vi "AT_Pro Main.vi"() -> ()   [LabVIEW 2018]
doc: "This template is for the Queued Message Handler design pattern.\n\nThe Event Handling Loop generates messages based on user interface actions.\n\nThe Message Handling Loop processes messages generated by the Event Handling Loop, or by other messages. The messages are string values, so new messages can be added easily to the Message Cases case structure in the Message Handling Loop. Each message cluster can also provide an optional value for Message Data, which is a variant that can be converted to whatever message-specific data is required."
uses:
  controls/AT_Pro UI Data.ctl
  <vilib>/DAQmx/read.llb/DAQmx Read (Analog 2D DBL NChan NSamp).vi
  support/Message Queue/Enqueue Message (Array).vi
  support/Message Queue/Enqueue Message (Single).vi
  <vilib>/DAQmx/miscellaneous.llb/DAQmx Fill In Error Info.vi
  <vilib>/Utility/error.llb/Error Cluster From Error Code.vi
  <vilib>/ErrorRing/Error Ring.xnode
  support/Message Queue/AT_Pro Message Queue.lvlib
  support/User Event - Stop/AT_Pro User Event - Stop.lvlib
panel:
  out "read buffer":string
  out "Waveform Graph":dbl[][](graph)
  in  "DAQmx Channel":tag="cDAQ1Mod4/ai17, cDAQ1Mod4/ai19"
  in  "COM Port":refnum<visa-resource-name>="COM8"
  in  "Stop Measure":bool
  in  "Start Measure":bool
  in  "Exit":bool
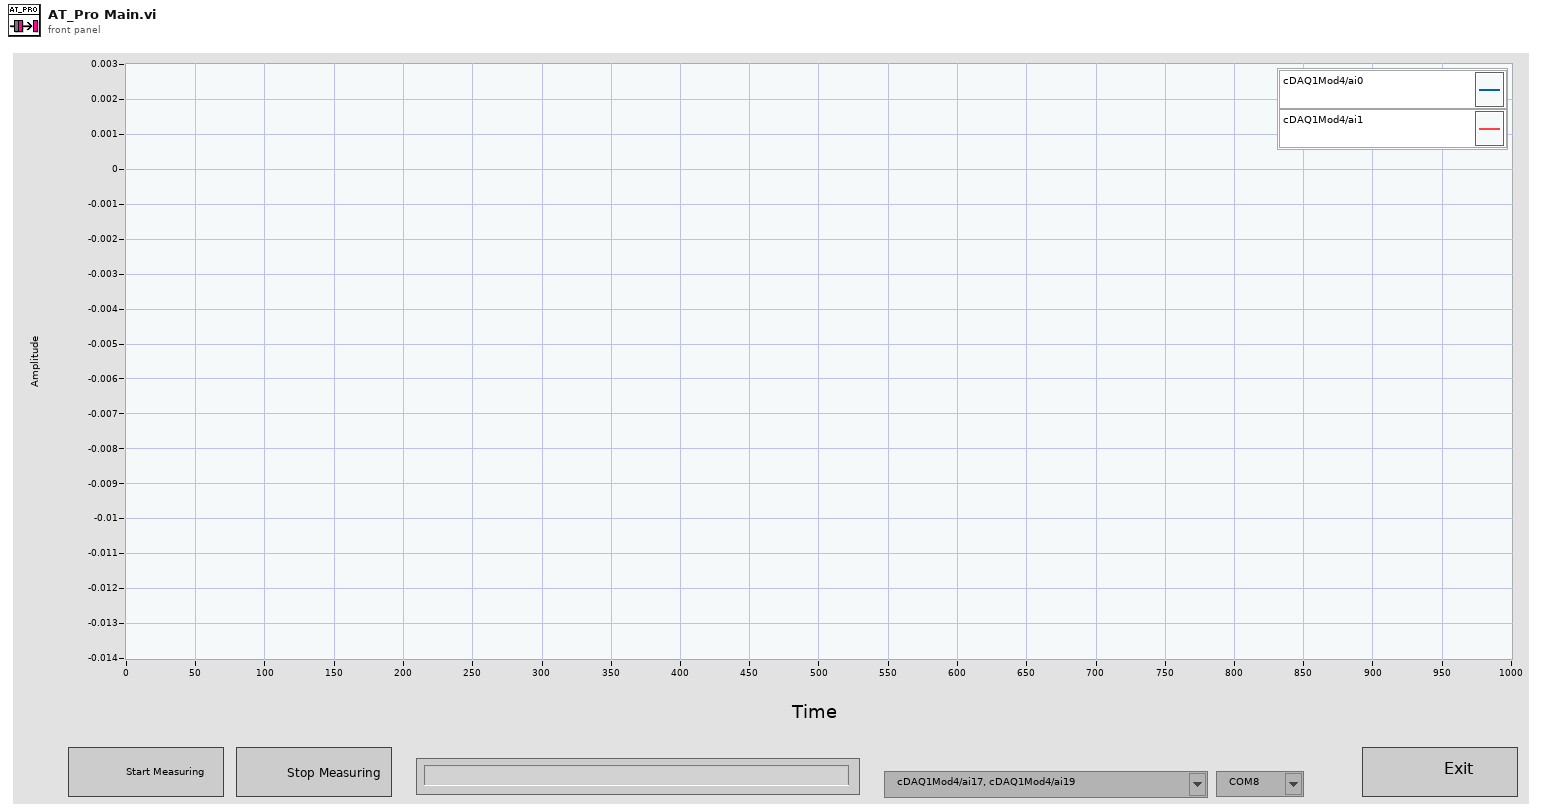
[diagram p1: front panel]
types:
  T1 = typedef "AT_Pro UI Data.ctl" = cluster{"Do Something Ref":refnum<vi>, "Do Something Else Ref":refnum<vi>, "Exit Button Ref":refnum<vi>, "Chart Refnum":refnum<vi>, "COM Port":refnum<visa-resource-name>, "DAQmx Ref":refnum<k21>}
  T2 = typedef "AT_Pro Message Queue.lvlib/All Message Queues.ctl" = cluster{"UI":refnum<queue>}
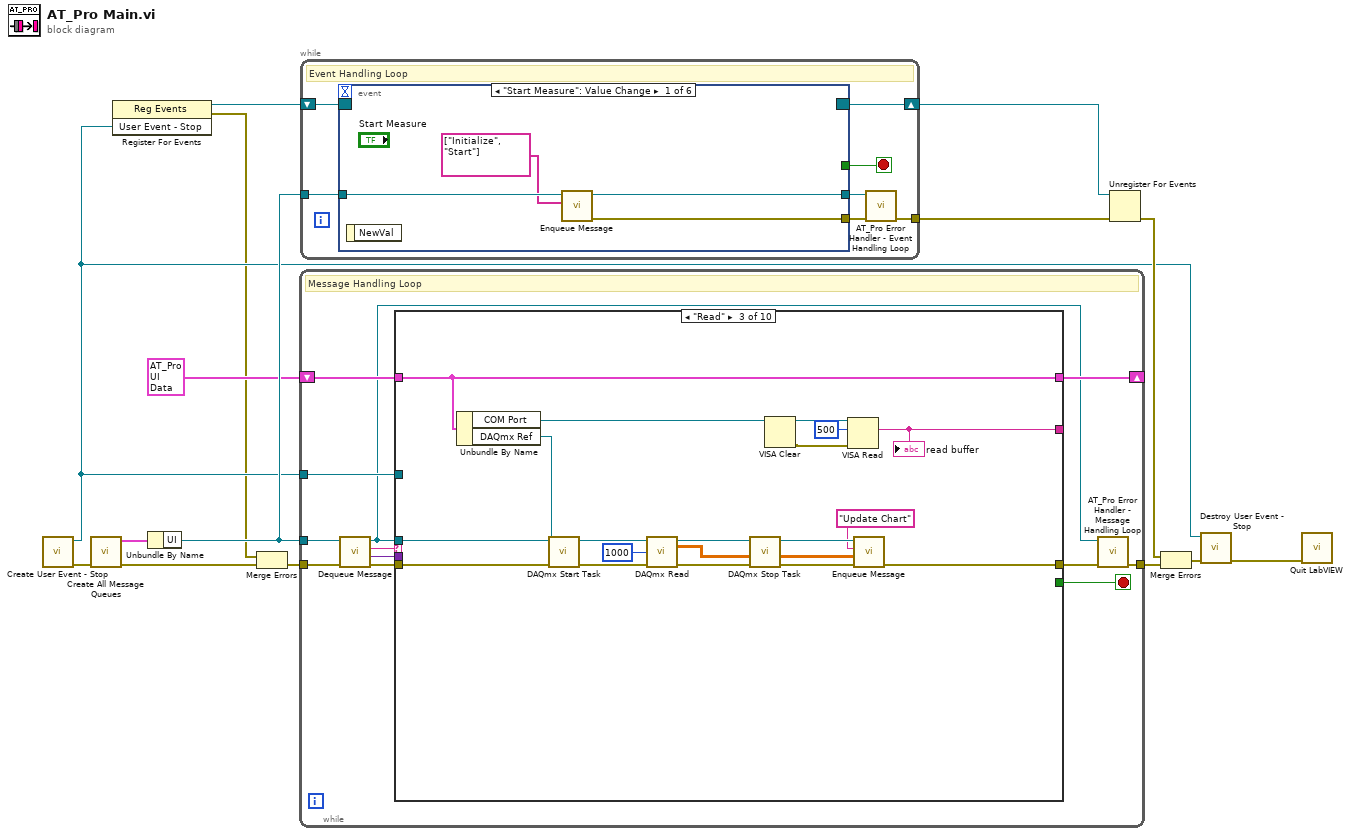
[diagram p0: block diagram]
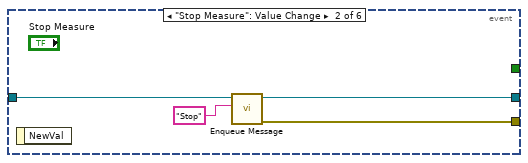
[diagram p2: hidden frame]
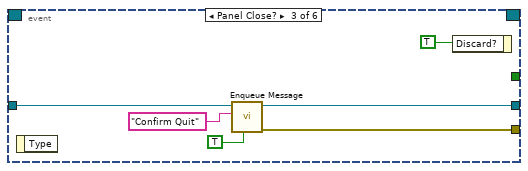
[diagram p3: hidden frame]
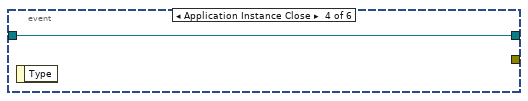
[diagram p4: hidden frame]
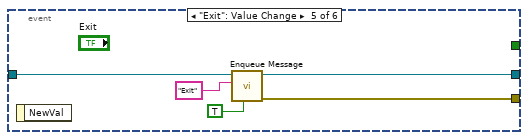
[diagram p5: hidden frame]
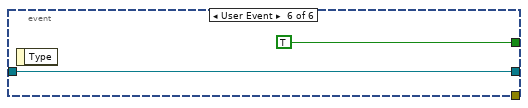
[diagram p6: hidden frame]
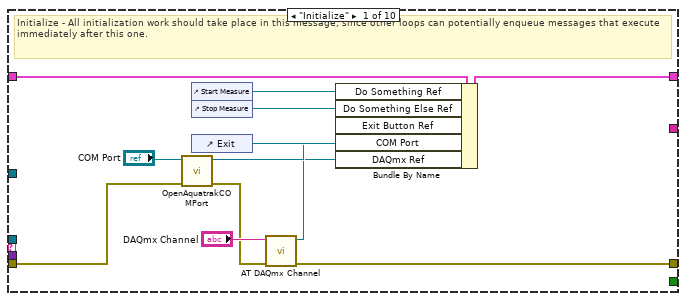
[diagram p7: hidden frame]
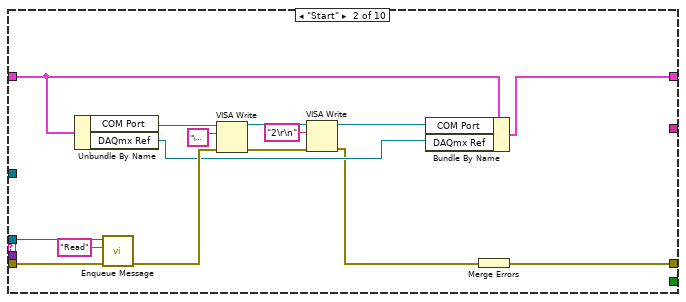
[diagram p8: hidden frame]
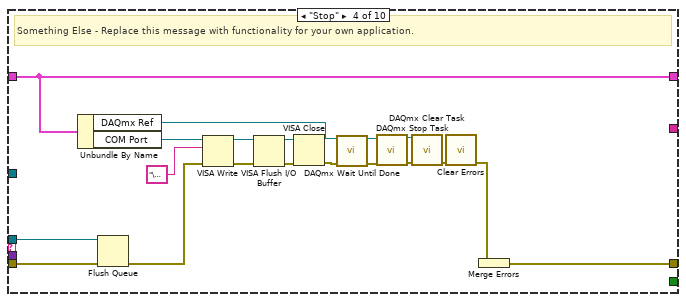
[diagram p9: hidden frame]
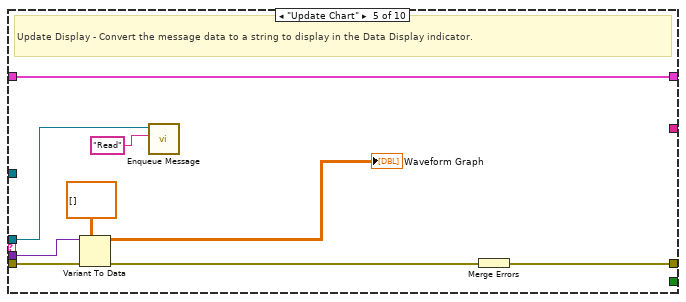
[diagram p10: hidden frame]
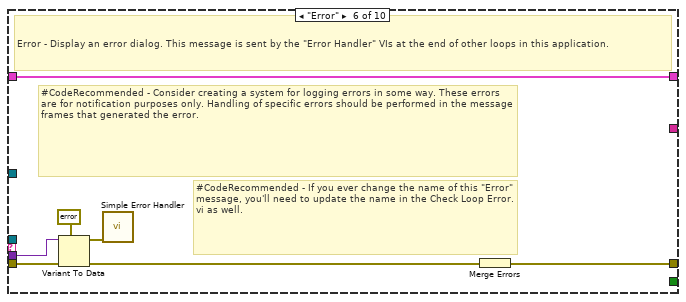
[diagram p11: hidden frame]
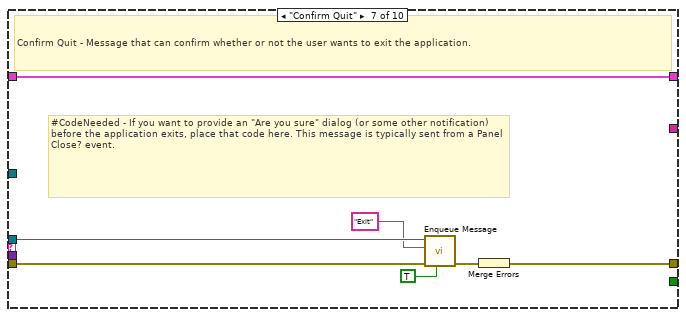
[diagram p12: hidden frame]
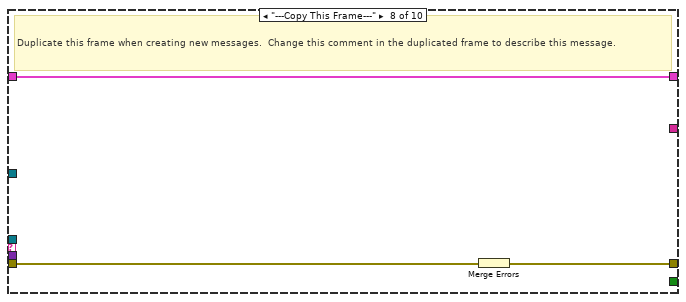
[diagram p13: hidden frame]
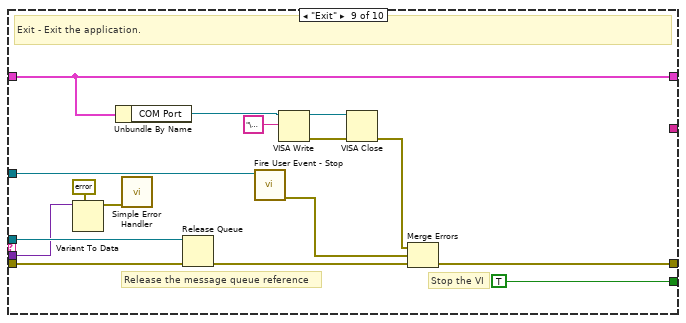
[diagram p14: hidden frame]
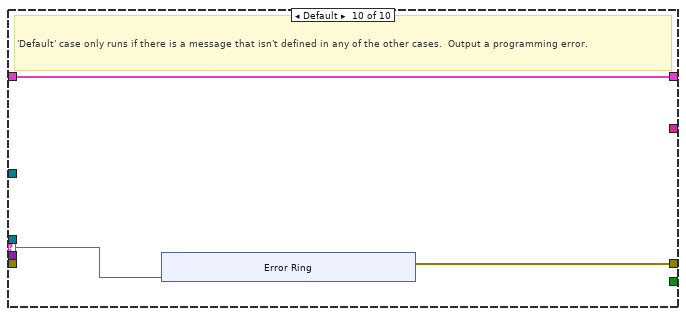
[diagram p15: hidden frame]
diagram:
  n1 = call "Create User Event - Stop.vi"() -> ("error out"=w11:errorcluster, "User Event - Stop"=w3:refnum<user-event>)  [unwired: 10 in]
  n2 = call "Create All Message Queues.vi"("error in (no error)"=w11) -> ("error out"=w15:errorcluster, "Message Queues out"=w14:T2)  [unwired: 9 in]
  n3 = register-events(w3) -> (reference out=w4:refnum<event-registration>, error out=w1:errorcluster)  [unwired: 2 in]
  n4 = Unbundle By Name(w14) -> ("UI"=w12:refnum<queue>)
  n5 = Merge Errors(w1, w15) -> (w2:errorcluster)
  n6 = while {
    tunnel: w12 -> [w19]
    shift-right: [w26] -> _
    shift-left: T1 {"Do Something Ref"=refnum, "Do Something Else Ref"=refnum, "Exit Button Ref"=refnum, "Chart Refnum"=refnum, "COM Port"="", "DAQmx Ref"=""} ("Data Cluster") -> [w27]
    tunnel: w3 -> [w24]
    tunnel: w2 -> [w23]
    tunnel: [w17] -> w13
    stop <- w25 stop-if-true
    # "Message Handling Loop"
    n7 = call "Dequeue Message.vi"("error in (no error)"=w23, "Message Queue"=w19) -> ("error out"=w22:errorcluster, "Message Data"=w20:variant, "Message"=w21:string, "dup Message Queue"=w18:refnum<queue>)  [unwired: 6 in]
    n8 = case "Message Cases" shown="\"Read\"" w21 {
      selector: w21 -> [_ _ _ _ _ _ _ _ _ w134]
      tunnel: w18 -> [_ w51 w69 w75 w94 _ w110 _ w133 _]
      tunnel: w22 -> [w33 w50 w62 w74 w98 w107 w114 w117 w129 _]
      tunnel: [w28 w54 w68 w91 w99 w101 w112 w115 w131 w135] -> w16
      tunnel: w27 -> [w39 w46 w72 w90 w100 w106 w113 w116 w125 w136]
      tunnel: [w38 w45 w72 w90 w100 w106 w113 w116 w125 w136] -> w26
      tunnel: [_ _ _ _ _ _ _ _ TRUE _] -> w25
      tunnel: w20 -> [_ _ _ _ w97 w105 _ _ w126 _]
      tunnel: w24 -> [_ _ _ _ _ _ _ _ w130 _]
      tunnel: [_ _ w66 _ _ _ _ _ _ _] -> _
      frame "Initialize" {
        # "Initialize - All initialization work should take place in this message, since other loops can potentially enqueue messages that execute immediately after this one."
        n9 = call "OpenAquatrakCOMPort.vi"("error in (no error)"=w33, "VISA Refnum in"="COM Port") -> ("error out"=w29:errorcluster, "VISA Refnum out"=w32:refnum<visa-resource-name>)  [unwired: 8 in]
        n10 = control-ref of="Start Measure"() -> (w37:refnum<vi>)
        n11 = control-ref of="Stop Measure"() -> (w36:refnum<vi>)
        n12 = control-ref of="Exit"() -> (w35:refnum<vi>)
        n13 = call "AT DAQmx Channel.vi"("error in"=w29, "DAQmx Physical Channel"="DAQmx Channel") -> ("error out"=w28:errorcluster, "Refnum out"=w30:refnum<k21>)  [unwired: 8 in]
        n14 = Bundle By Name(cluster=w39, "Do Something Ref"=w37, "Do Something Else Ref"=w36, "Exit Button Ref"=w35, "COM Port"=w32, "DAQmx Ref"=w30) -> (w38:T1)
      }
      frame "Start" {
        n15 = Unbundle By Name(w46) -> ("COM Port"=w53:refnum<visa-resource-name>, "DAQmx Ref"=w47:refnum<k21>)
        n16 = call-poly "Enqueue Message.vi"("error in (no error)"=w50, "Message"="Read", "Message Queue"=w51) -> ("error out"=w48:errorcluster)  [unwired: 7 in, 1 out]
        n17 = VISA Write(VISA resource name=w53, write buffer="\u001b", error in (no error)=w48) -> (VISA resource name out=w43:refnum<visa-resource-name>, error out=w42:errorcluster)  [unwired: 1 out]
        n18 = VISA Write(VISA resource name=w43, write buffer="2\r\n", error in (no error)=w42) -> (VISA resource name out=w41:refnum<visa-resource-name>, error out=w40:errorcluster)  [unwired: 1 out]
        n19 = Bundle By Name(cluster=w46, "COM Port"=w41, "DAQmx Ref"=w47) -> (w45:T1)
        n20 = Merge Errors(w40) -> (w54:errorcluster)
      }
      frame "Read" {
        n21 = Unbundle By Name(w72) -> ("COM Port"=w58:refnum<visa-resource-name>, "DAQmx Ref"=w64:refnum<k21>)
        n22 = call <vilib>:"DAQmx Start Task.vi"("task/channels in"=w64, "error in"=w62) -> ("task out"=w63:refnum<k21>, "error out"=w61:errorcluster)  [unwired: 12 in]
        n23 = call-poly <vilib>:"DAQmx Read.vi"("task/channels in"=w63, "number of samples per channel"=1000, "error in"=w61) -> ("task out"=w59:refnum<k21>, "data"=w70:dbl[][], "error out"=w60:errorcluster)  [unwired: 10 in]
        n24 = call <vilib>:"DAQmx Stop Task.vi"("task/channels in"=w59, "error in"=w60) -> ("error out"=w56:errorcluster)  [unwired: 12 in, 1 out]
        n25 = VISA Clear(VISA resource name=w58) -> (VISA resource name out=w57:refnum<visa-resource-name>, error out=w55:errorcluster)  [unwired: 1 in]
        n26 = VISA Read(VISA resource name=w57, byte count=u32 500, error in (no error)=w55) -> (read buffer=w66:string)  [unwired: 3 out]
        "read buffer" <- w66
        n27 = call-poly "Enqueue Message.vi"("error in (no error)"=w56, "Message Data"=w70, "Message"="Update Chart", "Message Queue"=w69) -> ("error out"=w68:errorcluster)  [unwired: 6 in, 1 out]
      }
      frame "Stop" {
        # "Something Else - Replace this message with functionality for your own application."
        n28 = Unbundle By Name(w90) -> ("DAQmx Ref"=w79:refnum<k21>, "COM Port"=w83:refnum<visa-resource-name>)
        n29 = Flush Queue(queue=w75, error in (no error)=w74) -> (error out=w73:errorcluster)  [unwired: 2 out]
        n30 = VISA Write(VISA resource name=w83, write buffer="\u001b", error in (no error)=w73) -> (VISA resource name out=w82:refnum<visa-resource-name>, error out=w81:errorcluster)  [unwired: 1 out]
        n31 = VISA Flush I/O Buffer(VISA resource name=w82, error in (no error)=w81) -> (VISA resource name out=w87:refnum<visa-resource-name>, error out=w88:errorcluster)  [unwired: 1 in]
        n32 = VISA Close(VISA resource name=w87, error in (no error)=w88) -> (error out=w78:errorcluster)
        n33 = call <vilib>:"DAQmx Wait Until Done.vi"("task/channels in"=w79, "error in"=w78) -> ("task out"=w77:refnum<k21>, "error out"=w76:errorcluster)  [unwired: 12 in]
        n34 = call <vilib>:"DAQmx Stop Task.vi"("task/channels in"=w77, "error in"=w76) -> ("task out"=w86:refnum<k21>, "error out"=w89:errorcluster)  [unwired: 12 in]
        n35 = call <vilib>:"DAQmx Clear Task.vi"("task in"=w86, "error in"=w89) -> ("error out"=w85:errorcluster)  [unwired: 13 in]
        n36 = call <vilib>:"Clear Errors.vi"("error in (no error)"=w85) -> ("error out"=w84:errorcluster)  [unwired: 5 in, 1 out]
        n37 = Merge Errors(w84) -> (w91:errorcluster)
      }
      frame "Update Chart" {
        # "Update Display - Convert the message data to a string to display in the Data Display indicator."
        n38 = Variant To Data(error in=w98, type=dbl[][] [] ("data"), Variant=w97) -> (data=→"Waveform Graph":dbl[][], error out=w96:errorcluster)
        n39 = call-poly "Enqueue Message.vi"("Message"="Read", "Message Queue"=w94) -> ()  [unwired: 8 in, 2 out]
        n40 = Merge Errors(w96) -> (w99:errorcluster)
      }
      frame "Error" {
        # "#CodeRecommended - If you ever change the name of this \"Error\" message, you'll need to update the name in the Check Loop Error.vi as well."
        # "#CodeRecommended - Consider creating a system for logging errors in some way. These errors are for notification purposes only. Handling of specific errors should be performed in the message frames that generated the error."
        # "Error - Display an error dialog. This message is sent by the \"Error Handler\" VIs at the end of other loops in this application."
        n41 = Variant To Data(error in=w107, type=errorcluster {"status"=FALSE, "code"=0, "source"=""} ("error constant"), Variant=w105) -> (data=w103:errorcluster, error out=w102:errorcluster)
        n42 = call <vilib>:"Simple Error Handler.vi"("error in (no error)"=w103) -> ()  [unwired: 4 in, 5 out]
        n43 = Merge Errors(w102) -> (w101:errorcluster)
      }
      frame "Confirm Quit" {
        # "#CodeNeeded - If you want to provide an \"Are you sure\" dialog (or some other notification) before the application exits, place that code here. This message is typically sent from a Panel Close? event."
        # "Confirm Quit - Message that can confirm whether or not the user wants to exit the application."
        n44 = call-poly "Enqueue Message.vi"("Priority Message? (F)"=TRUE, "error in (no error)"=w114, "Message"="Exit", "Message Queue"=w110) -> ("error out"=w111:errorcluster)  [unwired: 6 in, 1 out]
        n45 = Merge Errors(w111) -> (w112:errorcluster)
      }
      frame "---Copy This Frame---" {
        # "Duplicate this frame when creating new messages.  Change this comment in the duplicated frame to describe this message."
        n46 = Merge Errors(w117) -> (w115:errorcluster)
      }
      frame "Exit" {
        # "Stop the VI"
        # "Release the message queue reference"
        # "Exit - Exit the application."
        n47 = Variant To Data(type=errorcluster {"status"=FALSE, "code"=0, "source"=""} ("error constant"), Variant=w126) -> (data=w127:errorcluster)  [unwired: 1 in, 1 out]
        n48 = Unbundle By Name(w125) -> ("COM Port"=w121:refnum<visa-resource-name>)
        n49 = call <vilib>:"Simple Error Handler.vi"("error in (no error)"=w127) -> ()  [unwired: 4 in, 5 out]
        n50 = Release Queue(queue=w133, error in (no error)=w129) -> (error out=w124:errorcluster)  [unwired: 1 in, 2 out]
        n51 = call "Fire User Event - Stop.vi"("User Event - Stop"=w130) -> ("error out"=w122:errorcluster)  [unwired: 10 in]
        n52 = VISA Write(VISA resource name=w121, write buffer="\u001b") -> (VISA resource name out=w120:refnum<visa-resource-name>, error out=w119:errorcluster)  [unwired: 1 in, 1 out]
        n53 = VISA Close(VISA resource name=w120, error in (no error)=w119) -> (error out=w123:errorcluster)
        n54 = Merge Errors(w123, w122, w124) -> (w131:errorcluster)
      }
      frame Default {
        # "'Default' case only runs if there is a message that isn't defined in any of the other cases.  Output a programming error."
        n55 = xnode "Error Ring"("parameter 0"=w134) -> ("error out"=w135:errorcluster)
      }
    }
    n56 = call "AT_Pro Error Handler - Message Handling Loop.vi"("error in (no error)"=w16, "Message Queue"=w18) -> ("dup error in"=w17:errorcluster)  [unwired: 8 in, 1 out]
  }
  n57 = while {
    tunnel: w12 -> [w150]
    shift-right: [w148] -> w8
    shift-left: w4 -> [w149]
    tunnel: [w144] -> w5
    stop <- w146 stop-if-true
    # "Event Handling Loop"
    n58 = event shown="[0] \"Start Measure\": Value Change" {
      selector: w149 -> [_ _ _ _ _ _]
      dyn-events: [_ _ _ _ _ _] -> w148
      timeout: _ -> [_ _ _ _ _ _]
      tunnel: [_ _ _ _ _ TRUE ("Discard?")] -> w146
      tunnel: w150 -> [w154 w158 w163 w165 w170 w172]
      tunnel: [w152 w155 w162 _ w169 _] -> w147
      tunnel: [w153 w157 w161 w165 w168 w172] -> w145
      event "Start Measure": Value Change {
        n59 = event-data() -> ()  [unwired: 1 in, 1 out]
        n60 = call-poly "Enqueue Message.vi"("Message Array"=string[] ["Initialize", "Start"], "Message Queue"=w154) -> ("error out"=w152:errorcluster, "dup Message Queue"=w153:refnum<queue>)  [unwired: 8 in]
      }
      event "Stop Measure": Value Change {
        n61 = event-data() -> ()  [unwired: 1 in, 1 out]
        n62 = call-poly "Enqueue Message.vi"("Message"="Stop", "Message Queue"=w158) -> ("error out"=w155:errorcluster, "dup Message Queue"=w157:refnum<queue>)  [unwired: 8 in]
      }
      event Panel Close? {
        n63 = event-data() -> ()  [unwired: 1 in, 1 out]
        n64 = call-poly "Enqueue Message.vi"("Priority Message? (F)"=TRUE, "Message"="Confirm Quit", "Message Queue"=w163) -> ("error out"=w162:errorcluster, "dup Message Queue"=w161:refnum<queue>)  [unwired: 7 in]
        n65 = event-data("Discard?"=TRUE) -> ()  [unwired: 1 in, 1 out]
      }
      event Application Instance Close {
        n66 = event-data() -> ()  [unwired: 1 in, 1 out]
      }
      event "Exit": Value Change {
        n67 = event-data() -> ()  [unwired: 1 in, 1 out]
        n68 = call-poly "Enqueue Message.vi"("Priority Message? (F)"=TRUE, "Message"="Exit", "Message Queue"=w170) -> ("error out"=w169:errorcluster, "dup Message Queue"=w168:refnum<queue>)  [unwired: 7 in]
      }
      event User Event {
        n69 = event-data() -> ()  [unwired: 1 in, 1 out]
      }
    }
    n70 = call "AT_Pro Error Handler - Event Handling Loop.vi"("error in (no error)"=w147, "Message Queue"=w145) -> ("dup error in"=w144:errorcluster)  [unwired: 8 in, 1 out]
  }
  n71 = Unregister For Events(event registration refnum=w8, error in=w5) -> (error out=w9:errorcluster)
  n72 = Merge Errors(w9, w13) -> (w10:errorcluster)
  n73 = call "Destroy User Event - Stop.vi"("error in (no error)"=w10, "User Event - Stop"=w3) -> ("error out"=w6:errorcluster)  [unwired: 9 in]
  n74 = call "Quit LabVIEW.vi"("error in (no error)"=w6) -> ()  [unwired: 11 in]
